vi "YLabel1003.vi"   [LabVIEW 2013]
uses:
  <vilib>/Heliosphere Research LLC/Advanced Plotting Toolkit/api_annotations/LabelProperties.ctl
  <vilib>/Heliosphere Research LLC/Advanced Plotting Toolkit/properties/Text.ctl
  <vilib>/Heliosphere Research LLC/Advanced Plotting Toolkit/typedefs/PlotColor.ctl
  <vilib>/Heliosphere Research LLC/Advanced Plotting Toolkit/properties/Text_FontSize.ctl
  <vilib>/Heliosphere Research LLC/Advanced Plotting Toolkit/properties/Text_FontStyle.ctl
  <vilib>/Heliosphere Research LLC/Advanced Plotting Toolkit/Advanced Plotting Toolkit.lvlib
types:
  T1 = typedef "Advanced Plotting Toolkit.lvlib/Text_FontStyle.ctl" = enum16{"Automatic", "Normal", "Italic", "Bold"}
  T2 = typedef "Advanced Plotting Toolkit.lvlib/LabelProperties.ctl" = cluster{"Text":T3}
  T3 = typedef "Advanced Plotting Toolkit.lvlib/Text.ctl" = cluster{"Color":T4, "Background Color":T4, "Font Size (points)":T5, "Font Style":T1, "Rotation Angle":dbl}
  T4 = typedef "Advanced Plotting Toolkit.lvlib/PlotColor.ctl" = u32
  T5 = typedef "Advanced Plotting Toolkit.lvlib/Text_FontSize.ctl" = i32
  T6 = typedef "Advanced Plotting Toolkit.lvlib/PlotID.ctl" = i32
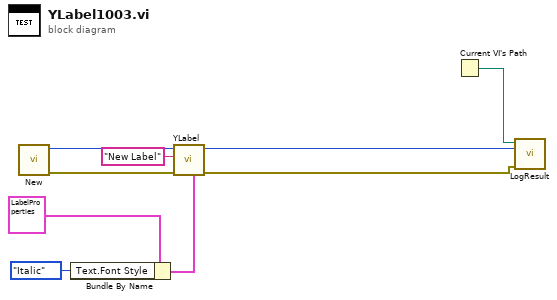
[diagram p0: block diagram]
diagram:
  n1 = call <vilib>:"New.vi"() -> ("error out"=w7:errorcluster, "Plot ID"=w8:T6)  [unwired: 10 in]
  n2 = Bundle By Name(cluster=T2 {"Text"={"Color"=2147483647, "Background Color"=2147483647, "Font Size (points)"=0, "Font Style"=enum."Automatic", "Rotation Angle"=nan}} ("Label Properties"), "Text.Font Style"=Text_FontStyle."Italic") -> (w2:T2)
  n3 = call <vilib>:"YLabel.vi"("Properties"=w2, "error in (no error)"=w7, "Label"="New Label" ("Title"), "Plot ID"=w8) -> ("error out"=w5:errorcluster, "Plot ID out"=w6:T6)  [unwired: 6 in]
  n4 = Current VI's Path() -> (path=w9:path)
  n5 = call "LogResult.vi"("Test Result"=w5, "Test Artifact"=w6, "VI Path"=w9) -> ()  [unwired: 9 in]
